vi "Create Refernce data.vi"(0 "Save Button":bool, 4 "Min_dist":dbl, 5 "vangle":dbl, 6 "layers":dbl, 7 "overlap":dbl, 8 "Interpolate":bool, 9 "height":dbl, 10 "width":dbl, 11 "increment":dbl) -> (1 "Reference":refnum<class "3D Plot Datatype.lvclass">[](xcontrol), 2 "3D Comet":refnum<class "3D Plot Datatype.lvclass">[](xcontrol))   [LabVIEW 2015]
uses:
  <vilib>/Math Plots/3D Math Plots/3D Scatter/3D Scatter XCtrl/3D Scatter.xctl
  <vilib>/Math Plots/3D Math Plots/3D Comet/3D Comet XCtrl/3D Comet.xctl
  Globals.vi
  <vilib>/Math Plots/3D Math Plots/3D Comet/3D Comet Datatype/Public/Plot Helper (Vector).vi
  <vilib>/Math Plots/3D Math Plots/3D Scatter/3D Scatter Datatype/Public/Plot Helper (Vector).vi
  <vilib>/Math Plots/3D Math Plots/3D Scatter/3D Scatter Datatype/3D Scatter Datatype.lvclass
  <vilib>/Math Plots/3D Math Plots/3D Comet/3D Comet Datatype/3D Comet Datatype.lvclass
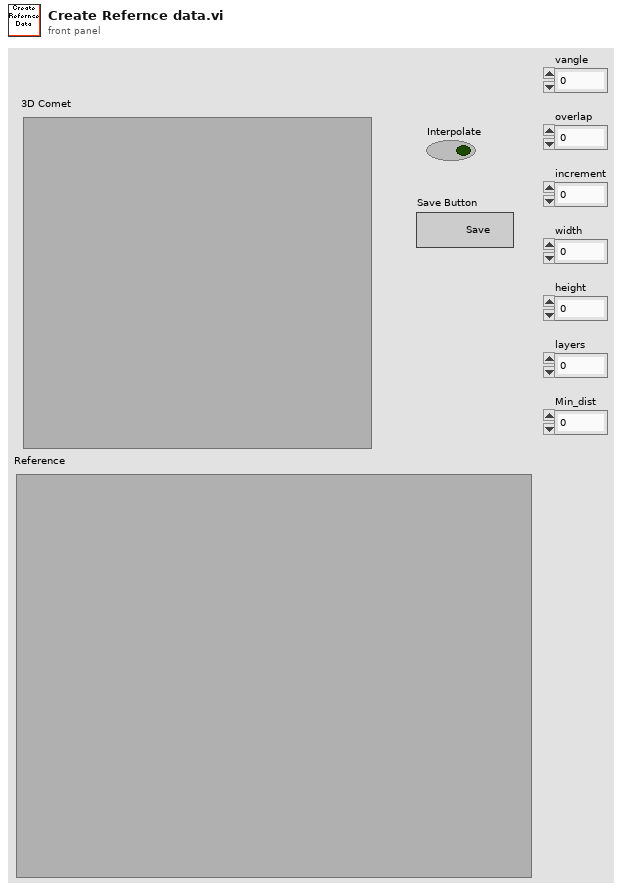
[diagram p1: front panel]
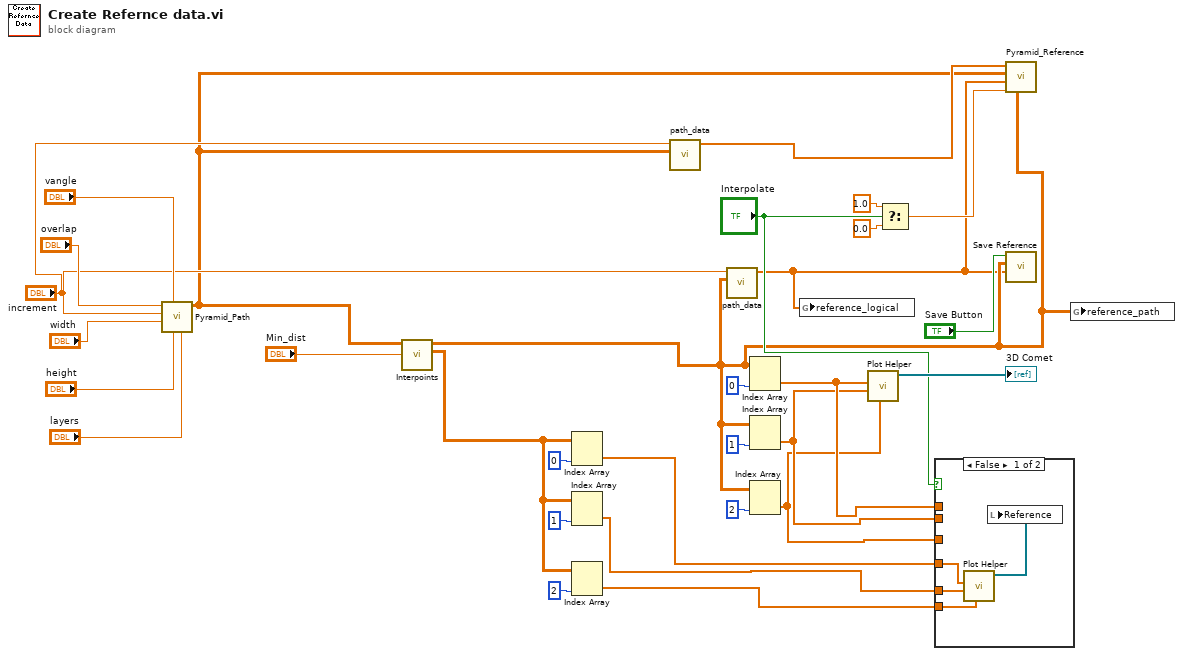
[diagram p0: block diagram]
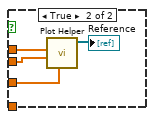
[diagram p2: hidden frame]
diagram:
  n1 = call "Pyramid_Path.vi"("layers"="layers", "height"="height", "vangle"="vangle", "width"="width", "increment"="increment", "overlap"="overlap") -> ("reference_corners"=w14:dbl[][])  [unwired: 5 in]
  n2 = call "Interpoints.vi"("Min_dist"="Min_dist", "reference_corners"=w14) -> ("Corners"=w18:dbl[][], "Reference path"=w2:dbl[][])  [unwired: 8 in]
  n3 = Index Array(array=w18, index (col)=0 ("disabled index (col)")) -> (element=w5:dbl[])  [unwired: 1 in]
  n4 = Index Array(array=w18, index (col)=1 ("disabled index (col)")) -> (element=w4:dbl[])  [unwired: 1 in]
  n5 = Index Array(array=w18, index (col)=2 ("disabled index (col)")) -> (element=w3:dbl[])  [unwired: 1 in]
  n6 = call "path_data.vi"("path in"=w14, "increment"="increment") -> ("path logical"=w15:dbl[])  [unwired: 9 in]
  n7 = call "path_data.vi"("path in"=w2, "increment"="increment") -> ("path logical"=w1:dbl[])  [unwired: 9 in]
  n8 = Index Array(array=w2, index (col)=0 ("disabled index (col)")) -> (element=w8:dbl[])  [unwired: 1 in]
  n9 = Index Array(array=w2, index (col)=1 ("disabled index (col)")) -> (element=w7:dbl[])  [unwired: 1 in]
  n10 = Index Array(array=w2, index (col)=2 ("disabled index (col)")) -> (element=w6:dbl[])  [unwired: 1 in]
  n11 = global write "Globals.vi" "reference_logical"(w1) -> ()
  n12 = call-poly <vilib>:"Plot Helper.vi"("z vector"=w6, "y vector"=w7, "x vector"=w8) -> ("3D Plot lvclass Array out"=→"3D Comet":refnum<class "3D Plot Datatype.lvclass">[])  [unwired: 3 in, 5 out]
  n13 = Select(t=1.0, s="Interpolate", f=0.0 ("t")) -> (s? t:f=w10:dbl)
  n14 = case shown="False" "Interpolate" {
    tunnel: w8 -> [_ w37]
    tunnel: w7 -> [_ w36]
    tunnel: w6 -> [_ w35]
    tunnel: w5 -> [w34 _]
    tunnel: w4 -> [w33 _]
    tunnel: w3 -> [w32 _]
    frame False {
      n15 = call-poly <vilib>:"Plot Helper.vi"("z vector"=w32, "y vector"=w33, "x vector"=w34) -> ("3D Plot lvclass Array out"=w31:refnum<class "3D Plot Datatype.lvclass">[])  [unwired: 3 in, 5 out]
      n16 = local write "Reference"(w31) -> ()
    }
    frame True {
      n17 = call-poly <vilib>:"Plot Helper.vi"("z vector"=w35, "y vector"=w36, "x vector"=w37) -> ("3D Plot lvclass Array out"=→"Reference":refnum<class "3D Plot Datatype.lvclass">[])  [unwired: 3 in, 5 out]
    }
  }
  n18 = call "Pyramid_Reference.vi"("Reference path"=w2, "interpolate"=w10, "Refernce_logical"=w1, "reference_corners"=w14, "corners_logical"=w15) -> ()  [unwired: 7 in]
  n19 = call "Save Reference.vi"("Refernce_logical"=w1, "Reference path"=w2, "Save Button"="Save Button") -> ()  [unwired: 9 in]
  n20 = global write "Globals.vi" "reference_path"(w2) -> ()
